vi "ImageDescription tag number.vi"() -> (0 "ImageDescription":u16=270)   [LabVIEW 2013, in "Tiff reader.lvlib"]
doc: "A constant that tells what tag number should be used for the metadata. (I have chosen 32781, the ImageID tag)"
uses:
  Tiff reader.lvlib
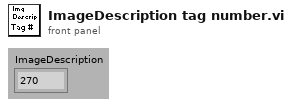
[diagram p1: front panel]
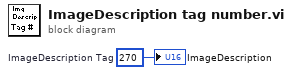
[diagram p0: block diagram]
diagram:
  w1 = u16 270  # ImageDescription Tag
  "ImageDescription" <- w1
